vi "collect_binstr.vi"(9 "Fraction":u8[](array[numeric]), 10 "Integer":u8[](array[numeric]), 11 "Sign":u8) -> (3 "String":string)   [LabVIEW 2025]
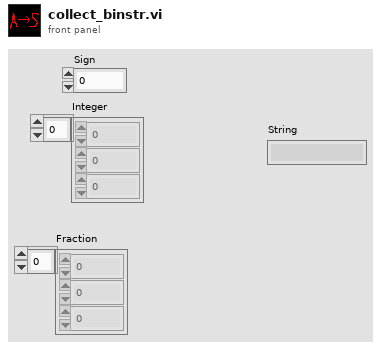
[diagram p1: front panel]
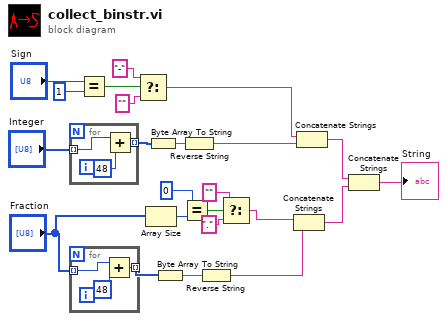
[diagram p0: block diagram]
diagram:
  n1 = for {
    tunnel: "Integer" -> [w26] mode=indexing
    tunnel: [w24] -> w9 mode=indexing
    n2 = Add(x=w26, y=u8 48) -> (x+y=w24:u8)
  }
  n3 = for {
    tunnel: "Fraction" -> [w29] mode=indexing
    tunnel: [w27] -> w8 mode=indexing
    n4 = Add(x=w29, y=u8 48) -> (x+y=w27:u8)
  }
  n5 = Equal?(x="Sign", y=u8 1) -> (x = y?=w21:bool)
  n6 = Select(t="-", s=w21, f="") -> (s? t:f=w18:string)
  n7 = Array Size(array="Fraction") -> (size(s)=w6:i32)
  n8 = Byte Array To String(unsigned byte array=w9) -> (string=w17:string)
  n9 = Byte Array To String(unsigned byte array=w8) -> (string=w15:string)
  n10 = Equal?(x=0, y=w6) -> (x = y?=w4:bool)
  n11 = Reverse String(1:w17) -> (0:w16:string)
  n12 = Reverse String(1:w15) -> (0:w14:string)
  n13 = Select(t="", s=w4, f="." ("string")) -> (s? t:f=w3:string)
  n14 = Concatenate Strings(w3, w14) -> (w12:string)
  n15 = Concatenate Strings(w18, w16) -> (w13:string)
  n16 = Concatenate Strings(w13, w12) -> (→"String":string)
